vi "Hexapod-Console.vi"(0 "CommCluster":T1={"PRAMMS-COMM"="Hp\u0000\u0002", "Signature"=1886544237, "MessageType"={["emtError", "emtAreYouThere", "emtAcknowledgment", "emtGetClientType", "emtClientType", "emtGetImageExposureTime", "emtSetImageExposureTime", "emtImageExposureTime", "emtGetOptimalExposureTime", "emtSetOptimalExposureTime", "emtOptimalExposureTime", "emtGetImageEMGain", "emtSetImageEMGain", "emtImageEMGain", "emtGetFPGACtrl", "emtSetFPGACtrl", "emtFPGACtrl", "emtGetImageWidth", "emtSetImageWidth", "emtImageWidth", "emtGetImageHeight", "emtSetImageHeight", "emtImageHeight", "emtGetImageBinning", "emtSetImageBinning", "emtImageBinning", "emtGetImageDisplayFrameRate", "emtSetImageDisplayFrameRate", "emtImageDisplayFrameRate", "emtGetROIWidth", "emtSetROIWidth", "emtROIWidth", "emtGetROIHeight", "emtSetROIHeight", "emtROIHeight", "emtGetROIXOffset", "emtSetROIXOffset", "emtROIXOffset", "emtGetROIYOffset", "emtSetROIYOffset", "emtROIYOffset", "emtStartAcquisition", "mtStopAcquisition", "emtAcquisitionStarted", "emtAcquisitionStopped", "emtGetFalconImage", "emtFalconImage"], [1, 2, 3, 4, 5, 1001, 1101, 1201, 1002, 1102, 1202, 1003, 1103, 1203, 1004, 1104, 1204, 1005, 1105, 1205, 1006, 1106, 1206, 1007, 1107, 1207, 1008, 1108, 1208, 1009, 1109, 1209, 1010, 1110, 1210, 1011, 1111, 1211, 1012, 1112, 1212, 1130, 1131, 1150, 1151, 1070, 1270]}, "Hexapod-COMM"="Hp\u0000\u0002"}, 2 "ReferenceCluster":T4, 11 "TelescopeCLuster":T3, 13 "HexapodCluster":T2) -> ()   [LabVIEW 2011]
uses:
  Polymorphics/Num2littleEndian(DBL).vi
panel:
  in  "Numeric":dbl
  out "Stop":bool
  in  "LoadLUT":bool
  in  "Quit&Kill":bool
  in  "Quit&Save":bool
  in  "Vitesse [um/s]":dbl step=10.0 format="%.1f"
  in  "X-":bool
  in  "X+":bool
  in  "Y-":bool
  in  "Y+":bool
  out "Azimuth":dbl=35996.6916 caption="Déclinaison du Télescope" format="%.4f"
  out "Altitude":dbl=35996.6916 caption="Déclinaison du Télescope" format="%.4f"
  in  "LUTData":string[][](table) caption="Points de la LUT"
  in  "RAZ":bool
  in  "SavePoint":bool
  in  "Move":bool
  out "Pos V":dbl format="%.4f"
  out "Pos U":dbl format="%.4f"
  out "Pos Z":dbl format="%.4f"
  out "Pos Y":dbl format="%.4f"
  out "Pos X":dbl format="%.4f"
  in  "Axe V":dbl format="%.4f"
  in  "Axe U":dbl format="%.4f"
  in  "Axe Z":dbl format="%.4f"
  in  "Axe Y":dbl format="%.4f"
  in  "Axe X":dbl format="%.4f"
  # "Position Actuelle"
  # "Position Commandée"
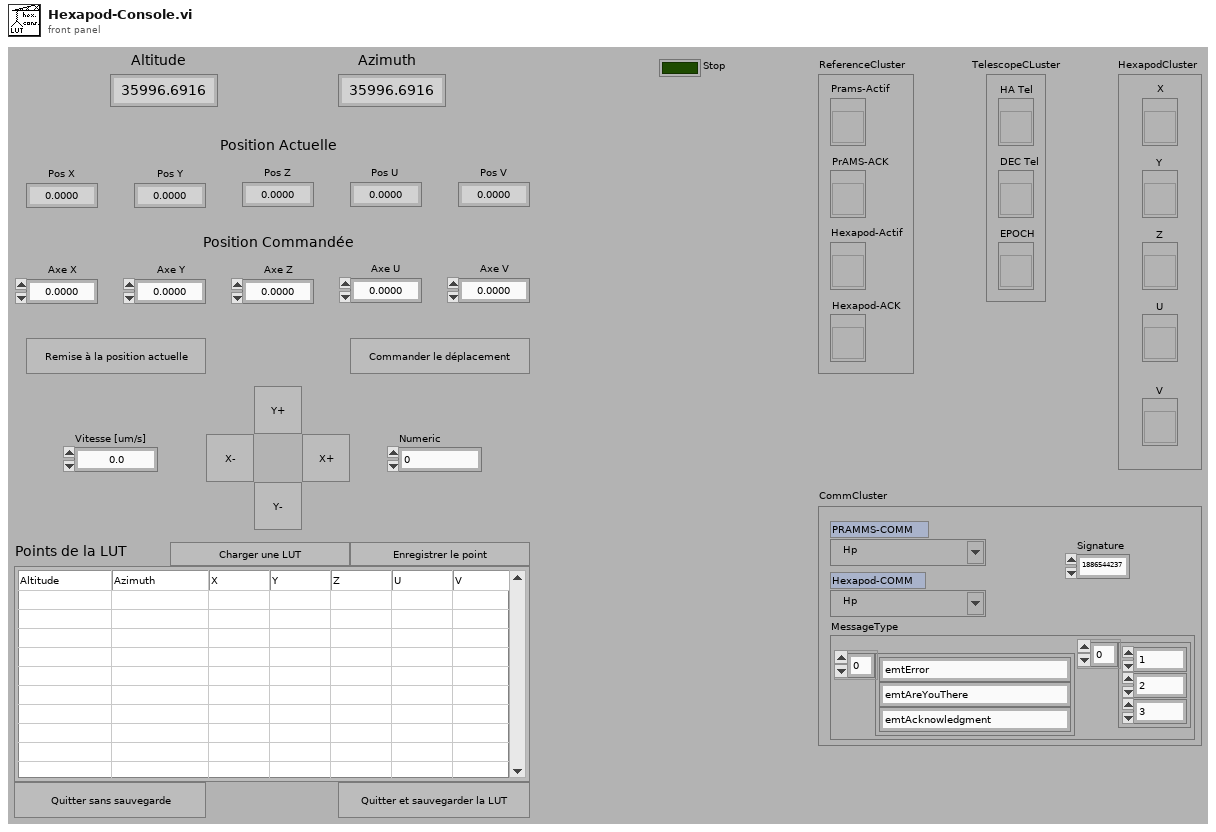
[diagram p1: front panel]
types:
  T1 = cluster{"PRAMMS-COMM":refnum<visa-resource-name>, "Signature":u32, "MessageType":cluster{string[], u32[]}, "Hexapod-COMM":refnum<visa-resource-name>}
  T2 = cluster{"X":refnum<vi>, "Y":refnum<vi>, "Z":refnum<vi>, "U":refnum<vi>, "V":refnum<vi>}
  T3 = cluster{"HA Tel":refnum<vi>, "DEC Tel":refnum<vi>, "EPOCH":refnum<vi>}
  T4 = cluster{"Prams-Actif":refnum<vi>, "PrAMS-ACK":refnum<vi>, "Hexapod-Actif":refnum<vi>, "Hexapod-ACK":refnum<vi>}
  T5 = enum8{"Enabled", "Disabled", "Disabled and Grayed Out"}
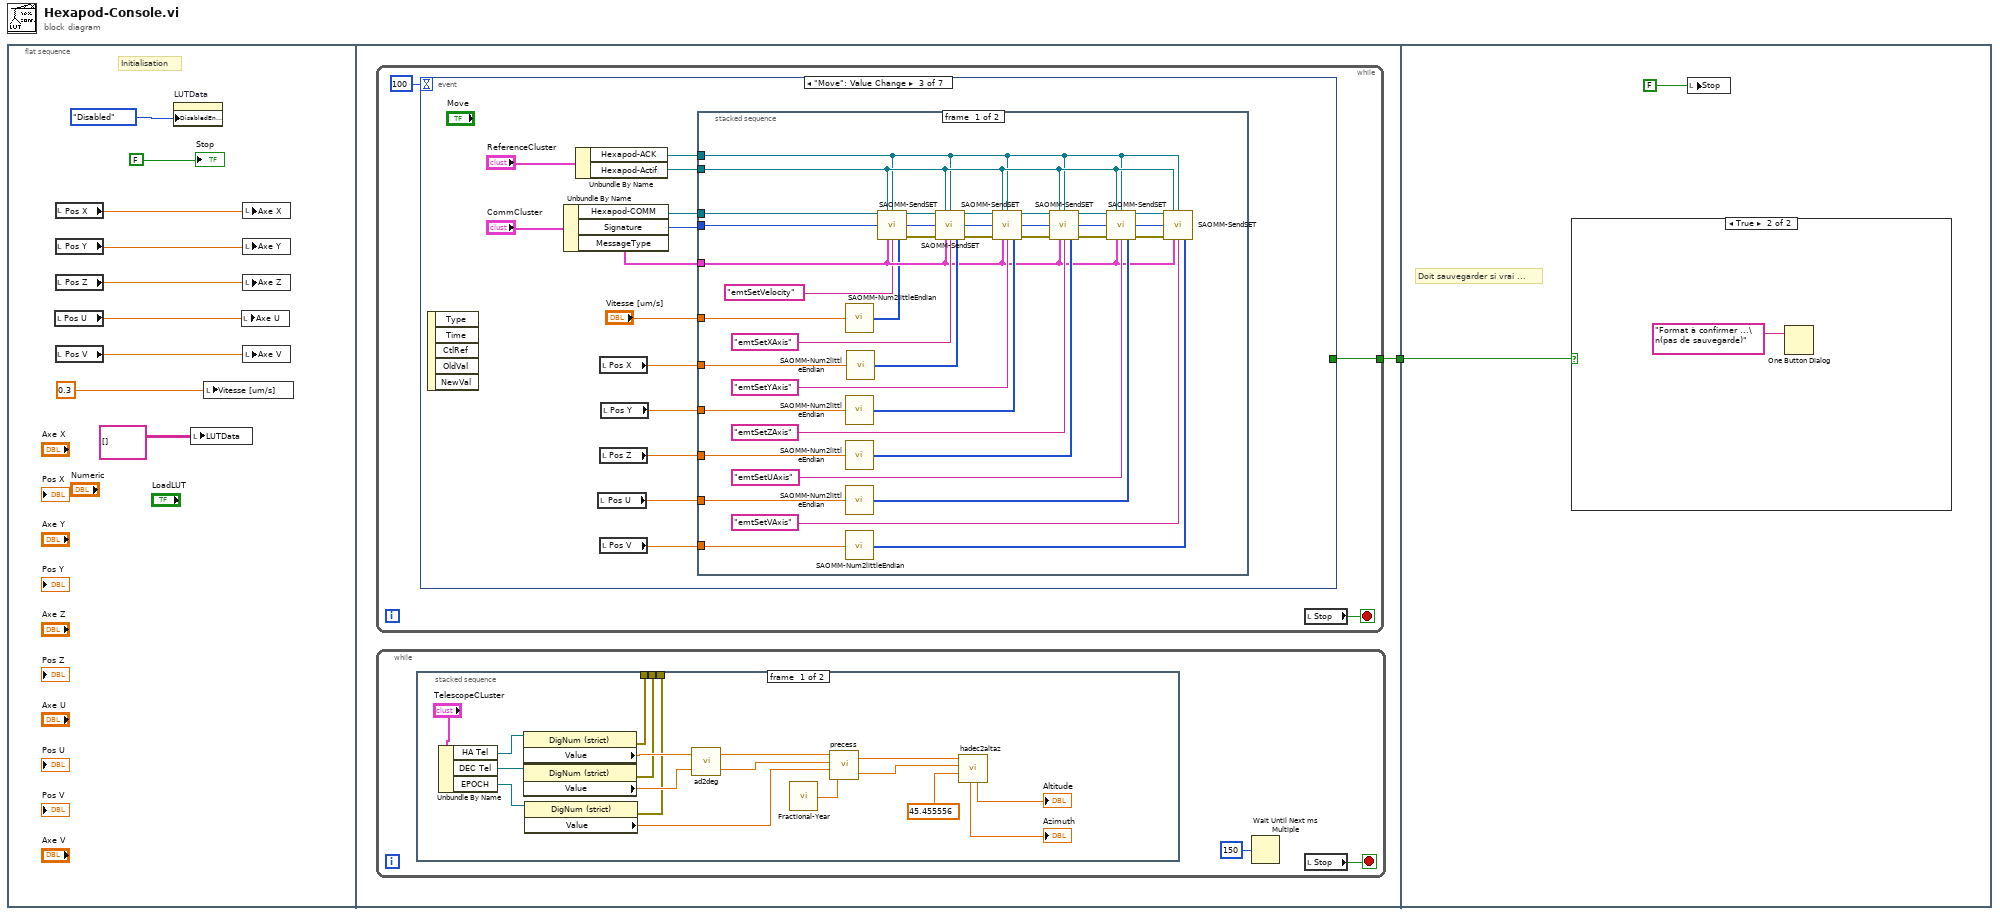
[diagram p0: block diagram]
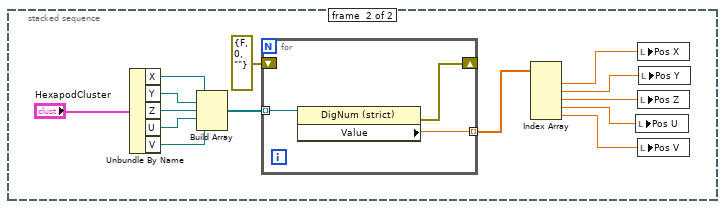
[diagram p2: hidden frame]
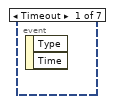
[diagram p3: hidden frame]
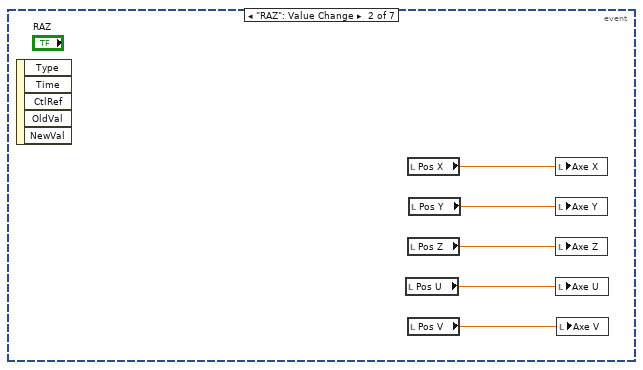
[diagram p4: hidden frame]
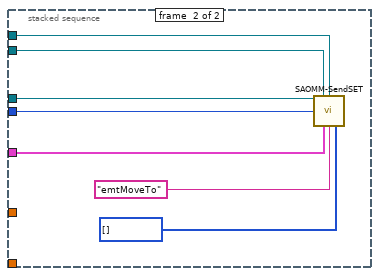
[diagram p5: hidden frame]
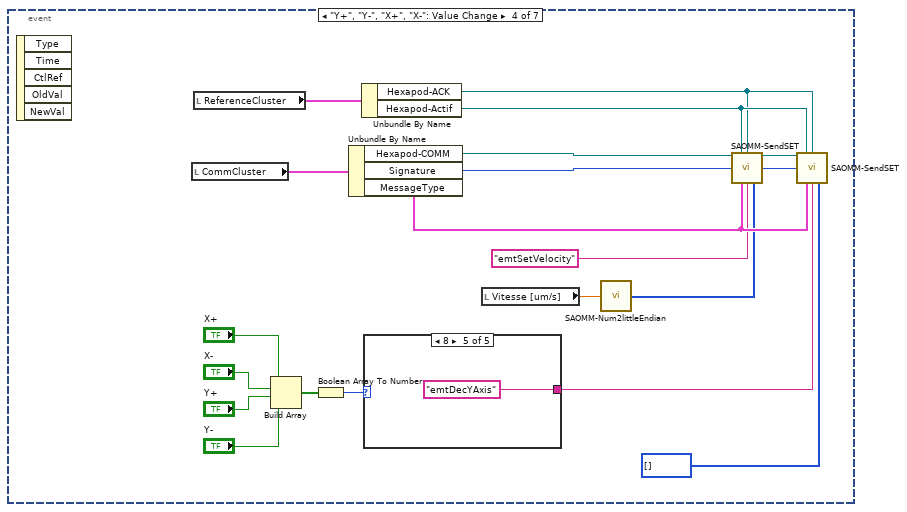
[diagram p6: hidden frame]
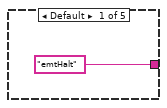
[diagram p7: hidden frame]
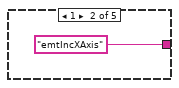
[diagram p8: hidden frame]
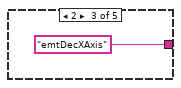
[diagram p9: hidden frame]
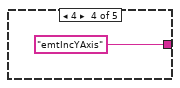
[diagram p10: hidden frame]
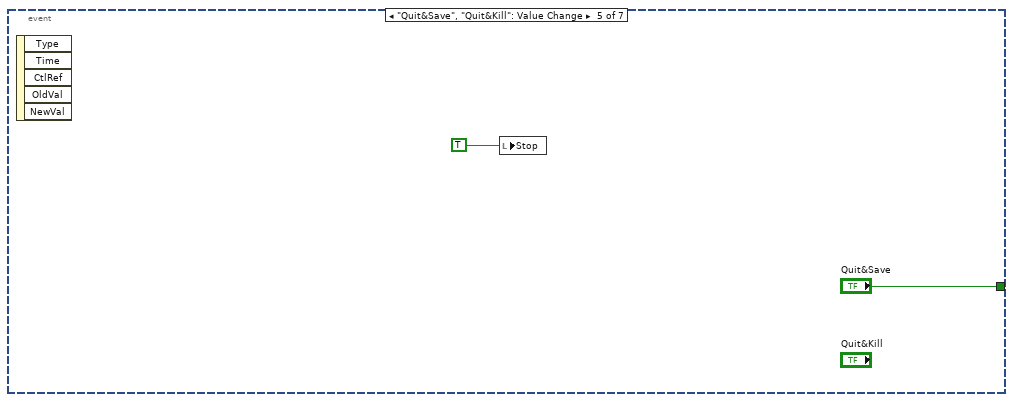
[diagram p11: hidden frame]
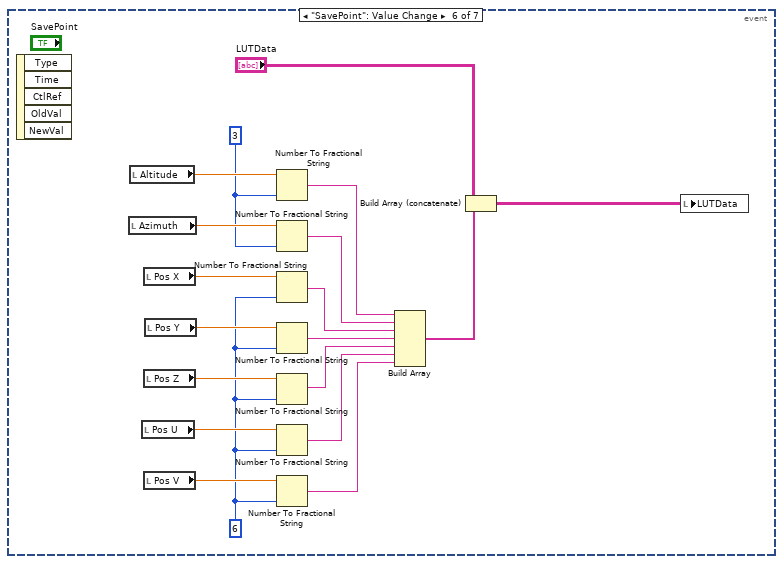
[diagram p12: hidden frame]
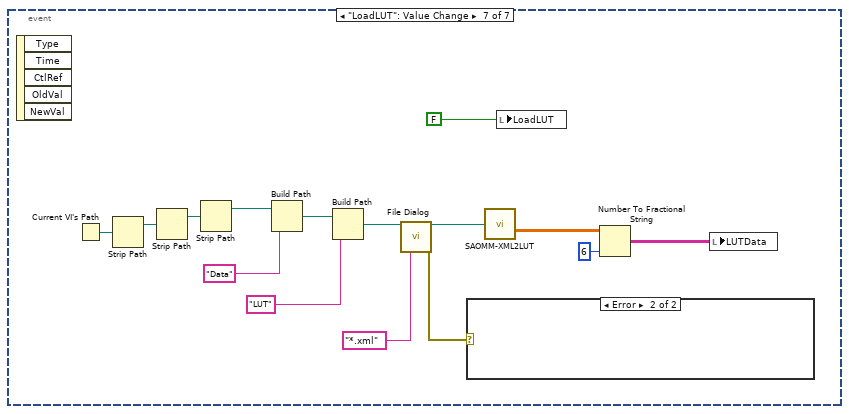
[diagram p13: hidden frame]
diagram:
  n1 = flat-sequence {
    tunnel: [w11] -> w1
    tunnel: w1 -> [w170]
    frame #0 {
      # "Initialisation"
      n2 = local read "Pos U"() -> (w5:dbl)
      n3 = local read "Pos X"() -> (w8:dbl)
      n4 = local read "Pos Y"() -> (w7:dbl)
      n5 = local read "Pos Z"() -> (w6:dbl)
      n6 = local read "Pos V"() -> (w4:dbl)
      n7 = property on="LUTData" class="Tbl (strict)"("DisabledEnum"=T5."Disabled" ("Disabled")) -> ()  [unwired: 2 in, 2 out]
      n8 = local write "LUTData"(string[][] [] ("LUTData")) -> ()
      n9 = local write "Vitesse [um/s]"(0.3 ("Vitesse [um/s]")) -> ()
      n10 = local write "Axe U"(w5) -> ()
      n11 = local write "Axe X"(w8) -> ()
      n12 = local write "Axe Y"(w7) -> ()
      n13 = local write "Axe Z"(w6) -> ()
      n14 = local write "Axe V"(w4) -> ()
      "Stop" <- FALSE ("Stop")
    }
    frame #1 {
      n15 = while {
        tunnel: [w49] -> w11
        stop <- w51 stop-if-true
        n16 = event shown="[2] \"Move\": Value Change" {
          selector: _ -> [_ _ _ _ _ _ _]
          dyn-events: _ -> [_ _ _ _ _ _ _]
          timeout: 100 -> [_ _ _ _ _ _ _]
          tunnel: [_ _ _ _ "Quit&Save" _ _] -> w49
          event Timeout {
            n17 = event-data() -> ()  [unwired: 1 in, 2 out]
          }
          event "RAZ": Value Change {
            n18 = event-data() -> ()  [unwired: 1 in, 5 out]
            n19 = local read "Pos U"() -> (w55:dbl)
            n20 = local read "Pos X"() -> (w52:dbl)
            n21 = local read "Pos Z"() -> (w54:dbl)
            n22 = local read "Pos V"() -> (w56:dbl)
            n23 = local read "Pos Y"() -> (w53:dbl)
            n24 = local write "Axe X"(w52) -> ()
            n25 = local write "Axe Y"(w53) -> ()
            n26 = local write "Axe Z"(w54) -> ()
            n27 = local write "Axe U"(w55) -> ()
            n28 = local write "Axe V"(w56) -> ()
          }
          event "Move": Value Change {
            n29 = event-data() -> ()  [unwired: 1 in, 5 out]
            n30 = Unbundle By Name("CommCluster") -> ("Hexapod-COMM"=w67:refnum<visa-resource-name>, "Signature"=w66:u32, "MessageType"=w68:cluster{string[], u32[]})
            n31 = Unbundle By Name("ReferenceCluster") -> ("Hexapod-ACK"=w63:refnum<vi>, "Hexapod-Actif"=w64:refnum<vi>)
            n32 = local read "Pos U"() -> (w59:dbl)
            n33 = local read "Pos X"() -> (w62:dbl)
            n34 = local read "Pos Z"() -> (w60:dbl)
            n35 = local read "Pos V"() -> (w58:dbl)
            n36 = local read "Pos Y"() -> (w61:dbl)
            n37 = stacked-sequence {
              tunnel: w67 -> [w79 w107]
              tunnel: w66 -> [w74 w106]
              tunnel: w68 -> [w73 w105]
              tunnel: w64 -> [w77 w104]
              tunnel: w63 -> [w76 w103]
              tunnel: w62 -> [w89 _]
              tunnel: w61 -> [w88 _]
              tunnel: w60 -> [w87 _]
              tunnel: w59 -> [w86 _]
              tunnel: w58 -> [w85 _]
              tunnel: "Vitesse [um/s]" -> [w70 _]
              frame #0 {
                n38 = call-poly "SAOMM-Num2littleEndian.vi"("Number"=w70) -> ("LiitleEndianedData"=w72:u8[])  [unwired: 14 in]
                n39 = call-poly "SAOMM-Num2littleEndian.vi"("Number"=w88) -> ("LiitleEndianedData"=w93:u8[])  [unwired: 14 in]
                n40 = call-poly "SAOMM-Num2littleEndian.vi"("Number"=w87) -> ("LiitleEndianedData"=w92:u8[])  [unwired: 14 in]
                n41 = call-poly "SAOMM-Num2littleEndian.vi"("Number"=w86) -> ("LiitleEndianedData"=w91:u8[])  [unwired: 14 in]
                n42 = call-poly "SAOMM-Num2littleEndian.vi"("Number"=w85) -> ("LiitleEndianedData"=w90:u8[])  [unwired: 14 in]
                n43 = call-poly "SAOMM-Num2littleEndian.vi"("Number"=w89) -> ("LiitleEndianedData"=w94:u8[])  [unwired: 14 in]
                n44 = call "SAOMM-SendSET.vi"("PRAMMS-COMM IN"=w79, "Active Refnum"=w77, "PrAMS-ACK"=w76, "Signature"=w74, "MessageType"=w73, "Active SET"="emtSetVelocity", "Value (little endianed byte array)"=w72) -> ("PRAMMS-COMM OUT"=w78:refnum<visa-resource-name>, "Error OUT"=w75:errorcluster)  [unwired: 5 in, 2 out]
                n45 = call "SAOMM-SendSET.vi"("PRAMMS-COMM IN"=w78, "Active Refnum"=w77, "PrAMS-ACK"=w76, "Signature"=w74, "Error IN"=w75, "MessageType"=w73, "Active SET"="emtSetXAxis", "Value (little endianed byte array)"=w94) -> ("PRAMMS-COMM OUT"=w102:refnum<visa-resource-name>, "Error OUT"=w98:errorcluster)  [unwired: 4 in, 2 out]
                n46 = call "SAOMM-SendSET.vi"("PRAMMS-COMM IN"=w102, "Active Refnum"=w77, "PrAMS-ACK"=w76, "Signature"=w74, "Error IN"=w98, "MessageType"=w73, "Active SET"="emtSetYAxis", "Value (little endianed byte array)"=w93) -> ("PRAMMS-COMM OUT"=w101:refnum<visa-resource-name>, "Error OUT"=w97:errorcluster)  [unwired: 4 in, 2 out]
                n47 = call "SAOMM-SendSET.vi"("PRAMMS-COMM IN"=w101, "Active Refnum"=w77, "PrAMS-ACK"=w76, "Signature"=w74, "Error IN"=w97, "MessageType"=w73, "Active SET"="emtSetZAxis", "Value (little endianed byte array)"=w92) -> ("PRAMMS-COMM OUT"=w100:refnum<visa-resource-name>, "Error OUT"=w96:errorcluster)  [unwired: 4 in, 2 out]
                n48 = call "SAOMM-SendSET.vi"("PRAMMS-COMM IN"=w100, "Active Refnum"=w77, "PrAMS-ACK"=w76, "Signature"=w74, "Error IN"=w96, "MessageType"=w73, "Active SET"="emtSetUAxis", "Value (little endianed byte array)"=w91) -> ("PRAMMS-COMM OUT"=w99:refnum<visa-resource-name>, "Error OUT"=w95:errorcluster)  [unwired: 4 in, 2 out]
                n49 = call "SAOMM-SendSET.vi"("PRAMMS-COMM IN"=w99, "Active Refnum"=w77, "PrAMS-ACK"=w76, "Signature"=w74, "Error IN"=w95, "MessageType"=w73, "Active SET"="emtSetVAxis", "Value (little endianed byte array)"=w90) -> ()  [unwired: 4 in, 4 out]
              }
              frame #1 {
                n50 = call "SAOMM-SendSET.vi"("PRAMMS-COMM IN"=w107, "Active Refnum"=w104, "PrAMS-ACK"=w103, "Signature"=w106, "MessageType"=w105, "Active SET"="emtMoveTo", "Value (little endianed byte array)"=u8[] []) -> ()  [unwired: 5 in, 4 out]
              }
            }
          }
          event "Y+", "Y-", "X+", "X-": Value Change {
            n51 = event-data() -> ()  [unwired: 1 in, 5 out]
            n52 = local read "CommCluster"() -> (w122:T1)
            n53 = local read "ReferenceCluster"() -> (w121:T4)
            n54 = Build Array("X+", "X-", "Y+", "Y-") -> (w128:bool[])
            n55 = Boolean Array To Number(Boolean array=w128) -> (number=w127:u32)
            n56 = Unbundle By Name(w122) -> ("Hexapod-COMM"=w114:refnum<visa-resource-name>, "Signature"=w113:u32, "MessageType"=w118:cluster{string[], u32[]})
            n57 = Unbundle By Name(w121) -> ("Hexapod-ACK"=w115:refnum<vi>, "Hexapod-Actif"=w116:refnum<vi>)
            n58 = case shown="8" w127 {
              tunnel: ["emtHalt" "emtIncXAxis" "emtDecXAxis" "emtIncYAxis" "emtDecYAxis"] -> w120
              frame Default {
                # "Aucun bouton n'a été appuyé"
              }
              frame 1 {
              }
              frame 2 {
              }
              frame 4 {
              }
              frame 8 {
              }
            }
            n59 = local read "Vitesse [um/s]"() -> (w112:dbl)
            n60 = call-poly "SAOMM-Num2littleEndian.vi"("Number"=w112) -> ("LiitleEndianedData"=w110:u8[])  [unwired: 14 in]
            n61 = call "SAOMM-SendSET.vi"("PRAMMS-COMM IN"=w114, "Active Refnum"=w116, "PrAMS-ACK"=w115, "Signature"=w113, "MessageType"=w118, "Active SET"="emtSetVelocity", "Value (little endianed byte array)"=w110) -> ("PRAMMS-COMM OUT"=w117:refnum<visa-resource-name>)  [unwired: 5 in, 3 out]
            n62 = call "SAOMM-SendSET.vi"("PRAMMS-COMM IN"=w117, "Active Refnum"=w116, "PrAMS-ACK"=w115, "Signature"=w113, "MessageType"=w118, "Active SET"=w120, "Value (little endianed byte array)"=u8[] []) -> ()  [unwired: 5 in, 4 out]
          }
          event "Quit&Save", "Quit&Kill": Value Change {
            n63 = event-data() -> ()  [unwired: 1 in, 5 out]
            n64 = local write "Stop"(TRUE ("Stop")) -> ()
          }
          event "SavePoint": Value Change {
            w146 = 6
            w147 = 3
            n65 = event-data() -> ()  [unwired: 1 in, 5 out]
            n66 = local read "Azimuth"() -> (w152:dbl)
            n67 = local read "Altitude"() -> (w153:dbl)
            n68 = local read "Pos U"() -> (w148:dbl)
            n69 = local read "Pos X"() -> (w151:dbl)
            n70 = local read "Pos Z"() -> (w149:dbl)
            n71 = local read "Pos V"() -> (w154:dbl)
            n72 = local read "Pos Y"() -> (w150:dbl)
            n73 = Number To Fractional String(number=w153, precision (6)=w147) -> (F-format string=w145:string)  [unwired: 2 in]
            n74 = Number To Fractional String(number=w152, precision (6)=w147) -> (F-format string=w144:string)  [unwired: 2 in]
            n75 = Number To Fractional String(number=w151, precision (6)=w146) -> (F-format string=w143:string)  [unwired: 2 in]
            n76 = Number To Fractional String(number=w150, precision (6)=w146) -> (F-format string=w142:string)  [unwired: 2 in]
            n77 = Number To Fractional String(number=w149, precision (6)=w146) -> (F-format string=w141:string)  [unwired: 2 in]
            n78 = Number To Fractional String(number=w148, precision (6)=w146) -> (F-format string=w140:string)  [unwired: 2 in]
            n79 = Number To Fractional String(number=w154, precision (6)=w146) -> (F-format string=w139:string)  [unwired: 2 in]
            n80 = Build Array(w145, w144, w143, w142, w141, w140, w139) -> (w138:string[])
            n81 = Build Array (concatenate)("LUTData", w138) -> (w136:string[][])
            n82 = local write "LUTData"(w136) -> ()
          }
          event "LoadLUT": Value Change {
            n83 = event-data() -> ()  [unwired: 1 in, 5 out]
            n84 = Current VI's Path() -> (path=w169:path)
            n85 = Strip Path(path=w169) -> (stripped path=w168:path)  [unwired: 1 out]
            n86 = Strip Path(path=w168) -> (stripped path=w161:path)  [unwired: 1 out]
            n87 = Strip Path(path=w161) -> (stripped path=w160:path)  [unwired: 1 out]
            n88 = Build Path(base path=w160, name or relative path="Data") -> (appended path=w159:path)
            n89 = Build Path(base path=w159, name or relative path="LUT") -> (appended path=w156:path)
            n90 = call "File Dialog"("start path"=w156, "pattern (all files)"="*.xml") -> ("selected path"=w167:path, "error out"=w162:errorcluster)  [unwired: 10 in, 2 out]
            n91 = case shown="Error" w162 {
              frame No Error {
              }
              frame Error {
              }
            }
            n92 = call "SAOMM-XML2LUT.vi"("Path"=w167) -> ("CompleteLUT"=w166:dbl[][])  [unwired: 13 in, 1 out]
            n93 = local write "LoadLUT"(FALSE ("LoadLUT")) -> ()
            n94 = Number To Fractional String(number=w166, precision (6)=i16 6) -> (F-format string=w164:string[][])  [unwired: 2 in]
            n95 = local write "LUTData"(w164) -> ()
          }
        }
        n96 = local read "Stop"() -> (w51:bool)
      }
      n97 = while {
        stop <- w13 stop-if-true
        n98 = stacked-sequence {
          tunnel: [w16 _] -> _
          tunnel: [w15 _] -> _
          tunnel: [w14 _] -> _
          frame #0 {
            n99 = Unbundle By Name("TelescopeCLuster") -> ("HA Tel"=w30:refnum<vi>, "DEC Tel"=w29:refnum<vi>, "EPOCH"=w25:refnum<vi>)
            n100 = property class="DigNum (strict)"(reference=w30) -> (error out=w16:errorcluster, "Value"=w22:dbl)  [unwired: 1 in, 1 out]
            n101 = property class="DigNum (strict)"(reference=w29) -> (error out=w15:errorcluster, "Value"=w21:dbl)  [unwired: 1 in, 1 out]
            n102 = property class="DigNum (strict)"(reference=w25) -> (error out=w14:errorcluster, "Value"=w18:dbl)  [unwired: 1 in, 1 out]
            n103 = call "ad2deg.vi"("DEC (sec)"=w21, "RA (sec)"=w22) -> ("DEC (°)"=w19:dbl, "RA (°)"=w20:dbl)
            n104 = call "Fractional-Year.vi"() -> ("Fractional Year"=w17:dbl)  [unwired: 15 in]
            n105 = call "precess.vi"("Eq2"=w17, "Eq1"=w18, "DEC 1"=w19, "RA 1"=w20) -> ("DEC 2"=w23:dbl, "RA 2"=w24:dbl)
            n106 = call "hadec2altaz.vi"("LAT"=45.455556, "DEC"=w23, "HA"=w24) -> ("Alt (theta)"=→"Altitude":dbl, "Az (phi)"=→"Azimuth":dbl)  [unwired: 4 in, 3 out]
          }
          frame #1 {
            n107 = Unbundle By Name("HexapodCluster") -> ("X"=w44:refnum<vi>, "Y"=w41:refnum<vi>, "Z"=w40:refnum<vi>, "U"=w42:refnum<vi>, "V"=w43:refnum<vi>)
            n108 = Build Array(w44, w41, w40, w42, w43) -> (w39:refnum<vi>[])
            n109 = for {
              tunnel: w39 -> [w48] mode=indexing
              shift-right: [w47] -> _
              shift-left: errorcluster {"status"=FALSE, "code"=0, "source"=""} ("error out") -> [_]
              tunnel: [w46] -> w37 mode=indexing
              n110 = property class="DigNum (strict)"(reference=w48) -> (error out=w47:errorcluster, "Value"=w46:dbl)  [unwired: 1 in, 1 out]
            }
            n111 = Index Array(array=w37) -> (element #1=w36:dbl, element #2=w35:dbl, element #3=w34:dbl, element #4=w33:dbl, element #5=w32:dbl)  [unwired: 5 in]
            n112 = local write "Pos U"(w33) -> ()
            n113 = local write "Pos X"(w36) -> ()
            n114 = local write "Pos Z"(w34) -> ()
            n115 = local write "Pos V"(w32) -> ()
            n116 = local write "Pos Y"(w35) -> ()
          }
        }
        n117 = Wait Until Next ms Multiple(millisecond multiple=u32 150) -> ()  [unwired: 1 out]
        n118 = local read "Stop"() -> (w13:bool)
      }
    }
    frame #2 {
      # "Doit sauvegarder si vrai ..."
      n119 = case shown="True" w170 {
        frame False {
        }
        frame True {
          n120 = One Button Dialog(message="Format à confirmer ...\n(pas de sauvegarde)") -> ()  [unwired: 1 in, 1 out]
        }
      }
      n121 = local write "Stop"(FALSE ("Stop")) -> ()
    }
  }
